vi "Module Init.vi"(8 "error in (no error)":errorcluster, 11 "Data Processor Module in":refnum<class "Data Processor Module.lvclass">) -> (0 "error out":errorcluster, 3 "Data Processor Module out":refnum<class "Data Processor Module.lvclass">)   [LabVIEW 2020, in "VolatusData.lvlib" / "Data Processor Module.lvclass"]
uses:
  Data Processor Module.lvclass
  Data Processor Module.lvclass/Data Processor Module.ctl
  Volatus/Module/Module.lvclass
  C:/dev/lv20CE/relink/lv-volatus/Volatus/Module/Module.lvclass
  C:/dev/lv20CE/relink/lv-volatus/VolatusData/Data Processor Module/Data Processor Module.lvclass
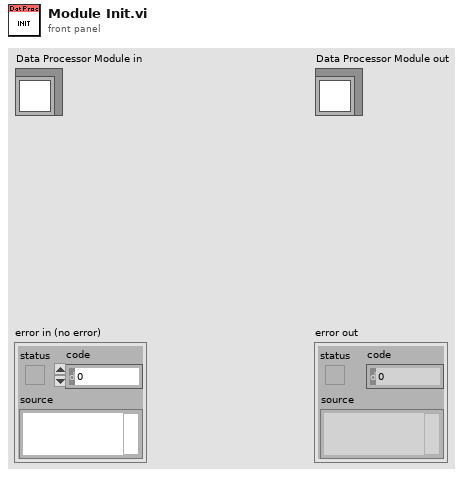
[diagram p1: front panel]
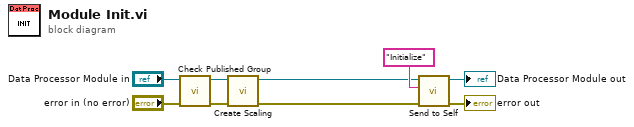
[diagram p0: block diagram]
diagram:
  n1 = call "Check Published Group.vi"("error in (no error)"="error in (no error)", "Data Processor Module in"="Data Processor Module in") -> ("error out"=w8:errorcluster, "Data Processor Module out"=w6:refnum<class "Data Processor Module.lvclass">)  [unwired: 8 in]
  n2 = call "Create Scaling.vi"("error in (no error)"=w8, "Data Processor Module in"=w6) -> ("error out"=w3:errorcluster, "Data Processor Module out"=w4:refnum<class "Data Processor Module.lvclass">)  [unwired: 8 in]
  n3 = call "Send to Self.vi"("error in (no error)"=w3, "Message ID"="Initialize", "Module in"=w4) -> ("error out"=→"error out":errorcluster, "Module out"=→"Data Processor Module out":refnum<class "Data Processor Module.lvclass">)  [unwired: 7 in]
